vi "F Dwf Analog Impedance Status Input.vi"(7 "pradian":dbl, 8 "error in (no error)":errorcluster, 9 "pgain":dbl, 10 "idxChannel":i32, 11 "hdwf":i32) -> (0 "error out":errorcluster, 1 "pgain out":dbl, 3 "function return":i32, 5 "pradian out":dbl)   [LabVIEW 2021, in "Olasdwf.lvlib"]
doc: "DWFAPI int FDwfAnalogImpedanceStatusInput(HDWF hdwf, int idxChannel, double *pgain, double *pradian);"
uses:
  Olasdwf.lvlib
  Windows/System32/dwf.dll
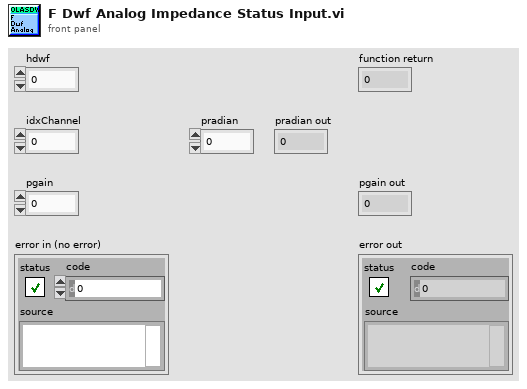
[diagram p1: front panel]
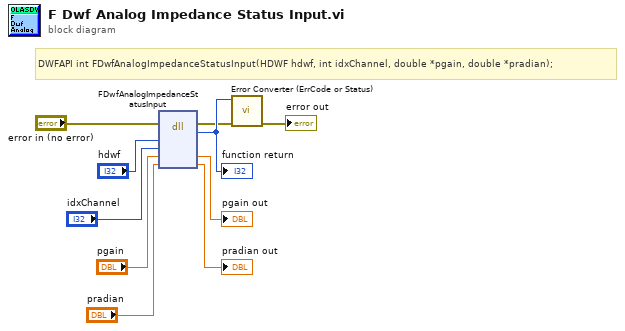
[diagram p0: block diagram]
diagram:
  # "DWFAPI int FDwfAnalogImpedanceStatusInput(HDWF hdwf, int idxChannel, double *pgain, double *pradian);"
  n1 = dll-call lib="/Windows/System32/dwf.*" fn="FDwfAnalogImpedanceStatusInput"(error in="error in (no error)", "hdwf"="hdwf", "idxChannel"="idxChannel", "pgain"="pgain", "pradian"="pradian") -> (error out=w2:errorcluster, w10:i32, "pgain"=→"pgain out":dbl, "pradian"=→"pradian out":dbl)  [unwired: 4 in, 1 out]
  "function return" <- w10
  n2 = call "Error Converter (ErrCode or Status).vi"("error in (no error)"=w2, "error code"=w10) -> ("error out"=→"error out":errorcluster)  [unwired: 9 in]
